vi "Host_GUI.vi"() -> ()   [LabVIEW 2017]
uses:
  <vilib>/Platform/TimedLoop/XDataNode/timing_clust.ctl
  <vilib>/Platform/TimedLoop/XDataNode/nitl_modes.ctl
  <vilib>/Platform/TimedLoop/XDataNode/wakeup.ctl
  <vilib>/Platform/TimedLoop/XDataNode/XDataNode.xnode
  <vilib>/FTP/NI_FTP.lvlib
  <vilib>/Platform/TimedLoop/XDataNode/XDNodeRunTimeDep.lvlib
panel:
  out "min index(es)":i32
  out "min value":dbl
  out "array":dbl[][](array[numeric])
  out "Enum":T1(ring)
  in  "Tab Control":T2(tab)
  in  "Initialization Parameters":T3={"W_b ini [rad/s]"=[0.0, 0.0, 0.0], "W ini [rad/s]"=[0.0, 0.0, 0.0], "altitude_ini(m)"=50.638, "lon_ini [º]"=-44.367775, "latd_ini [º]"=-2.3159948, "V_ini [m/s]"=[0.0, 0.0, 0.0], "Initial Euler Angles [deg]"=[0.0, 0.0, 0.0], "CFN-61G Enable"=FALSE, "Table enable"=FALSE, "DMARS Enable"=FALSE, "German TVA Enable"=FALSE, "Sim_Time [s]"=82.0, "Control Selection"=enum."Sim Control", "LOG Enable"=FALSE, "BR ACT enable"=FALSE} {"lon_ini [º]" format="%#_11g"; "latd_ini [º]" format="%#_10g"}
  in  "Simulation Parameters":T4={"Wind VelocityAzimuth [deg] "=0.0, "Wind Velocity Module [m/s]"=0.0, "Fe gain"=1.0, "Cnalpha gain"=1.0, "clp gain"=1.0, "cld gain"=1.0, "cmq gain"=1.0, "cnr gain"=1.0, "dl [º]"=0.0, "Nozzle misalignment yaw/pitch [º]"=[0.0, 0.0], "Nozzle eccentricity yaw/pitch [m]"=[], "Wind_Profile"=0} {"Wind_Profile" min=0 max=3 step=1; "Wind Velocity Module [m/s]" format="%#_13g"; "Wind VelocityAzimuth [deg]" format="%#_13g"}
  in  "Continuar":bool
  in  "stop":bool
  in  "Continuar":bool
  out "Table Monitor":T5(graph)
  out "OUTER":cluster{dbl, dbl, dbl} {"?" format="%1_6g"}
  out "INNER":cluster{dbl, dbl, dbl} {"?" format="%_6g"; "?" format="%#1_6g"}
  out "MIDDLE":cluster{dbl, dbl, dbl} {"?" format="%1_6g"}
  out "Euler Angles Simulation [deg]":T5(graph)
  in  "START_SIM":bool
  out "Sim_Stopped":bool
  in  "stop RT":bool
  out "Simulation time [s]":dbl
  out "Atitude":refnum<vi>(3d-picture)
  out "Altitude [m]":dbl
  out "Latitude/Longitude Sim [deg]":dbl[](array[numeric])
  out "Table ready":bool
  in  "Selector":enum16{"INNER", "MIDDLE", "OUTER"}(ring)=enum."OUTER"
  out "Euler Angles CFN [deg]":T5(graph)
  out "Euler Angles Diff (sim; INS)":cluster{dbl, dbl, dbl}
  out "Latitude/Longitude Ref [deg]":dbl[](array[numeric])
  out "Iteration Duration":i64
  out "Table Commands":T5(graph)
  in  "Selector 2":enum16{"INNER", "MIDDLE", "OUTER"}(ring)=enum."OUTER"
  out "Rates Sim [deg/s]":cluster{dbl, dbl, dbl}
  in  "Tab Control 2":T6(tab)
  out "Position":cluster{dbl[], dbl[]}[](graph)
  out "Velocity":cluster{dbl[], dbl[]}[](graph)
  out "Quaternions":cluster{dbl[], dbl[]}[](graph)
  out "Euler Angles":cluster{dbl[], dbl[]}[](graph)
  out "Body Rates":cluster{dbl[], dbl[]}[](graph)
  out "Body Accelerations":cluster{dbl[], dbl[]}[](graph)
  out "Malpha/ Mbeta":cluster{dbl[], dbl[]}[](graph)
  out "Angles of attack":cluster{dbl[], dbl[]}[](graph)
  out "ACT_b_angles":cluster{dbl[], dbl[]}[](graph)
  out "Oil Consumption":cluster{dbl[], dbl[]}(graph)
  out "Bending Moments":dbl[](graph)
  out "Guidance errors":cluster{dbl[], dbl[]}[](graph)
  out "Pos comparison":cluster{dbl[], dbl[]}[](graph)
  out "Euler Angles 2":cluster{dbl[], dbl[]}[](graph)
  out "file error":errorcluster
  # "POS"
  # "RATE"
  # "ACCEL"
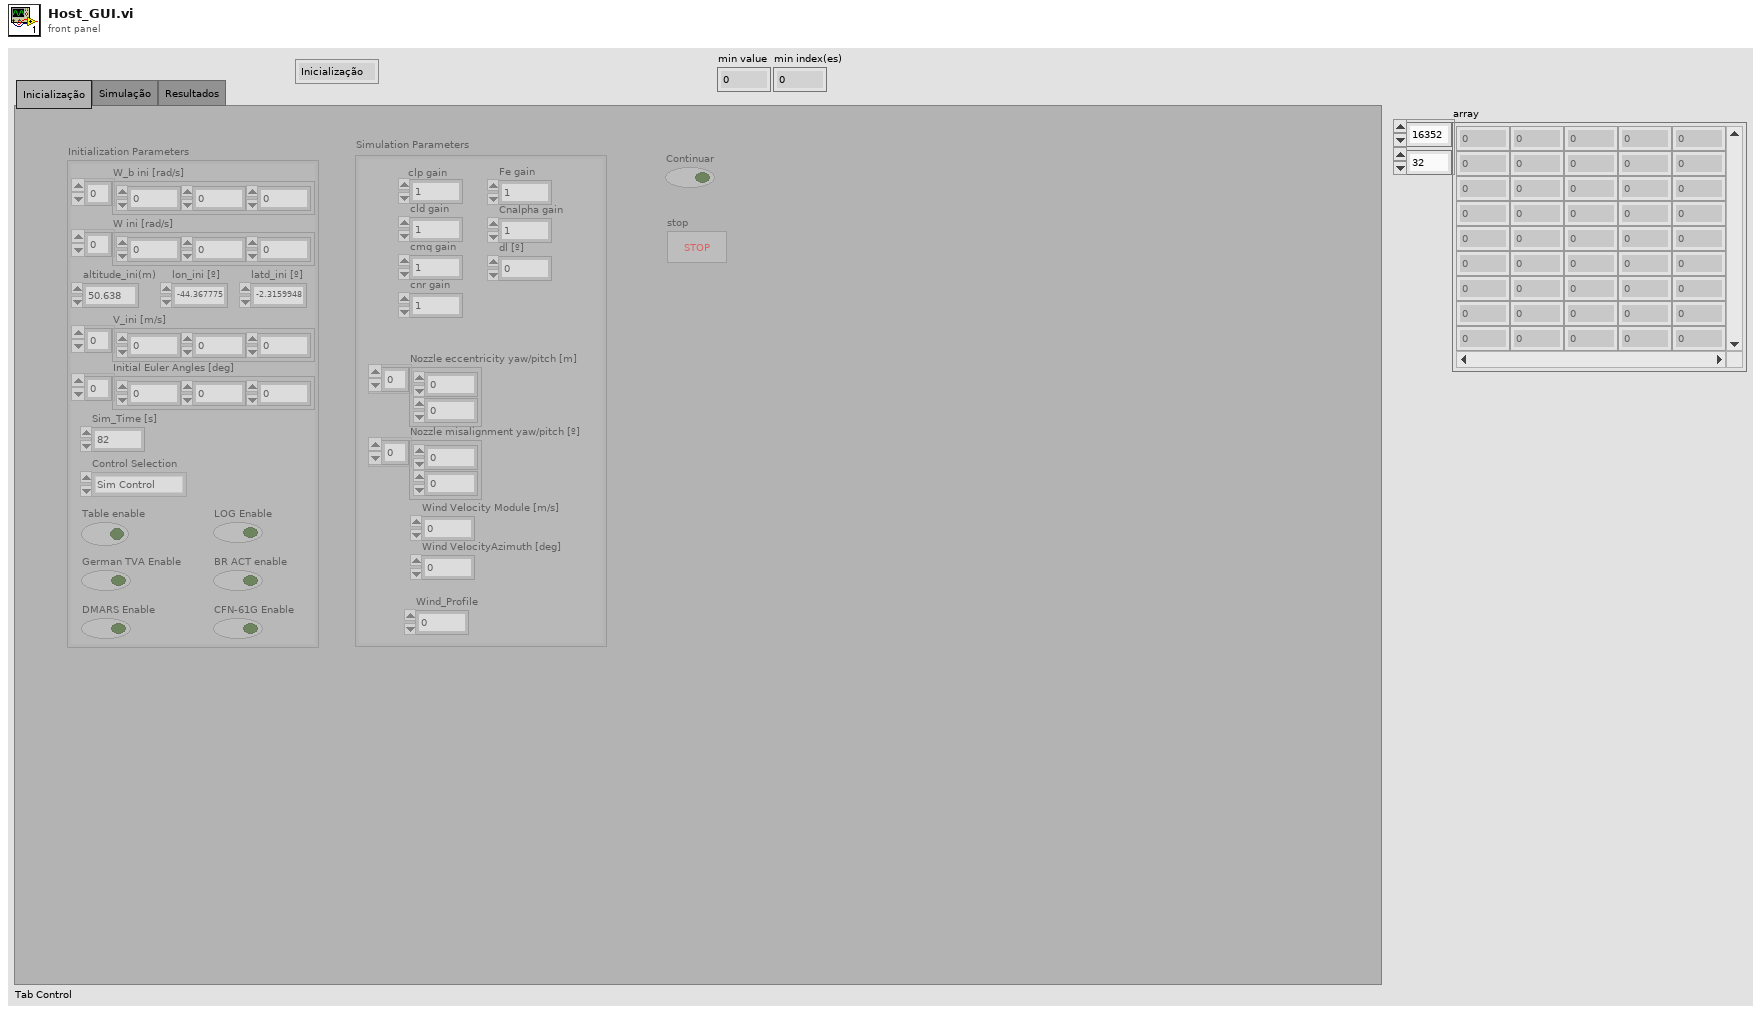
[diagram p1: front panel]
types:
  T1 = enum16{"Inicialização", "Simulação", "Resultados", "Finalizar RT"}
  T2 = enum32{"Inicialização", "Simulação", "Resultados"}
  T3 = cluster{"W_b ini [rad/s]":dbl[], "W ini [rad/s]":dbl[], "altitude_ini(m)":dbl, "lon_ini [º]":dbl, "latd_ini [º]":dbl, "V_ini [m/s]":dbl[], "Initial Euler Angles [deg]":dbl[], "CFN-61G Enable":bool, "Table enable":bool, "DMARS Enable":bool, "German TVA Enable":bool, "Sim_Time [s]":dbl, "Control Selection":enum16{"Constant", "TVA E-BOX", "Sim Control"}, "LOG Enable":bool, "BR ACT enable":bool}
  T4 = cluster{"Wind VelocityAzimuth [deg] ":dbl, "Wind Velocity Module [m/s]":dbl, "Fe gain":dbl, "Cnalpha gain":dbl, "clp gain":dbl, "cld gain":dbl, "cmq gain":dbl, "cnr gain":dbl, "dl [º]":dbl, "Nozzle misalignment yaw/pitch [º]":dbl[], "Nozzle eccentricity yaw/pitch [m]":dbl[], "Wind_Profile":i32}
  T5 = cluster{"Numeric":dbl, "Numeric":dbl, "Numeric":dbl}
  T6 = enum32{"Position", "Velocity", "Attitude Quaternions", "Attitude Euler Angles", "Body Rates", "Accel", "Malpha/ Mbeta", "AoA", "ACT_b angles", "Oil Consumption", "Bending Moments", "Guidance errors", "Position Comparison", "Attitude Comparison"}
  T7 = enum8{"Enabled", "Disabled", "Disabled and Grayed Out"}
  T8 = typedef "XDNodeRunTimeDep.lvlib/timing_clust.ctl" = cluster{"Expected End [f-1]":u64, "Actual End [f-1]":u64, "Finished Late? [f-1]":bool, "Expected End [i-1]":u64, "Actual End [i-1]":u64, "Finished Late? [i-1]":bool, "Expected Start [i]":u64, "Actual Start [i]":u64, "Expected Start [f]":u64, "Actual Start [f]":u64, "Source Name":string, "Structure Name":string, "Period":i64, "Deadline":i64, "Offset":i64, "Start":i64, "Priority":i32, "Timeout":i32, "Mode":T9, "Wakeup Reason":T10, "Error":errorcluster, "Source Type":string, "Secondary Source Type":string, "Global End Time":u64, "Global Start Time":u64, "Frame Duration":u64, "Iteration Duration":u64, "Assigned CPU":i32, "I/O Scan Engine Mode":u32}
  T9 = typedef "XDNodeRunTimeDep.lvlib/nitl_modes.ctl" = enum32{"No Change", "Process missed periods, maintain original phase", "Discard missed periods, maintain original phase", "Process missed periods, ignore original phase", "Discard missed periods, ignore original phase"}
  T10 = typedef "XDNodeRunTimeDep.lvlib/wakeup.ctl" = enum32{"Normal", "Aborted", "Asynchronous wakeup", "Timing source error", "Timed loop error", "Timeout"}
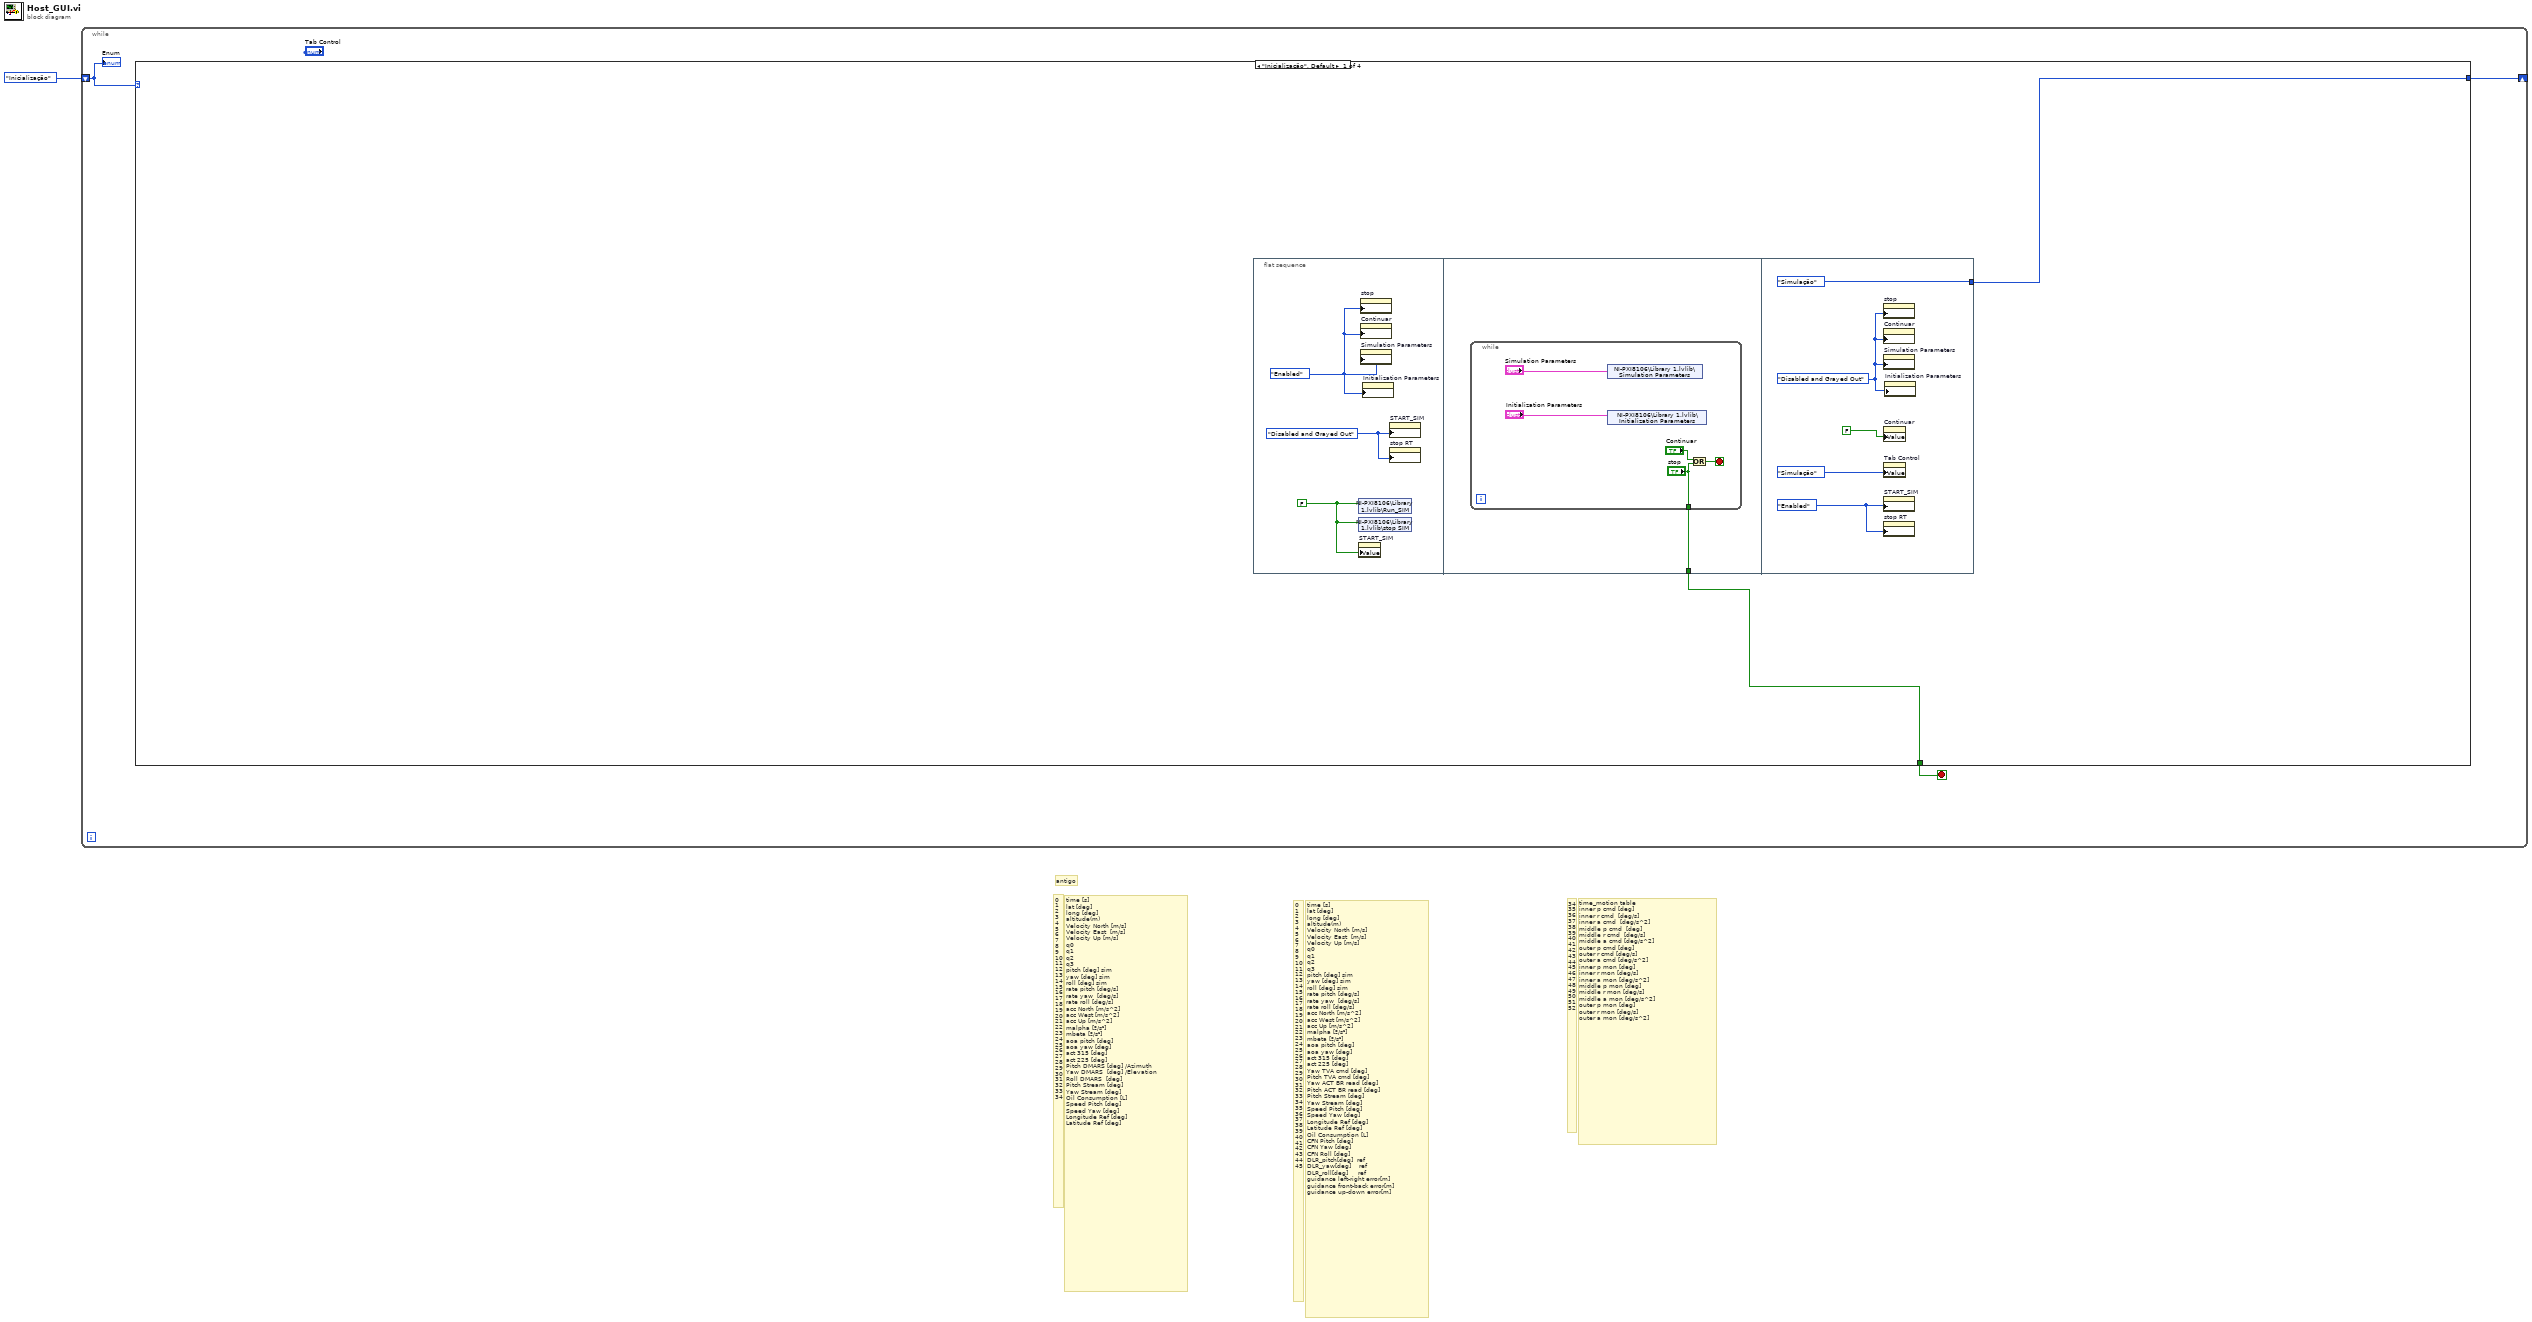
[diagram p0: block diagram]
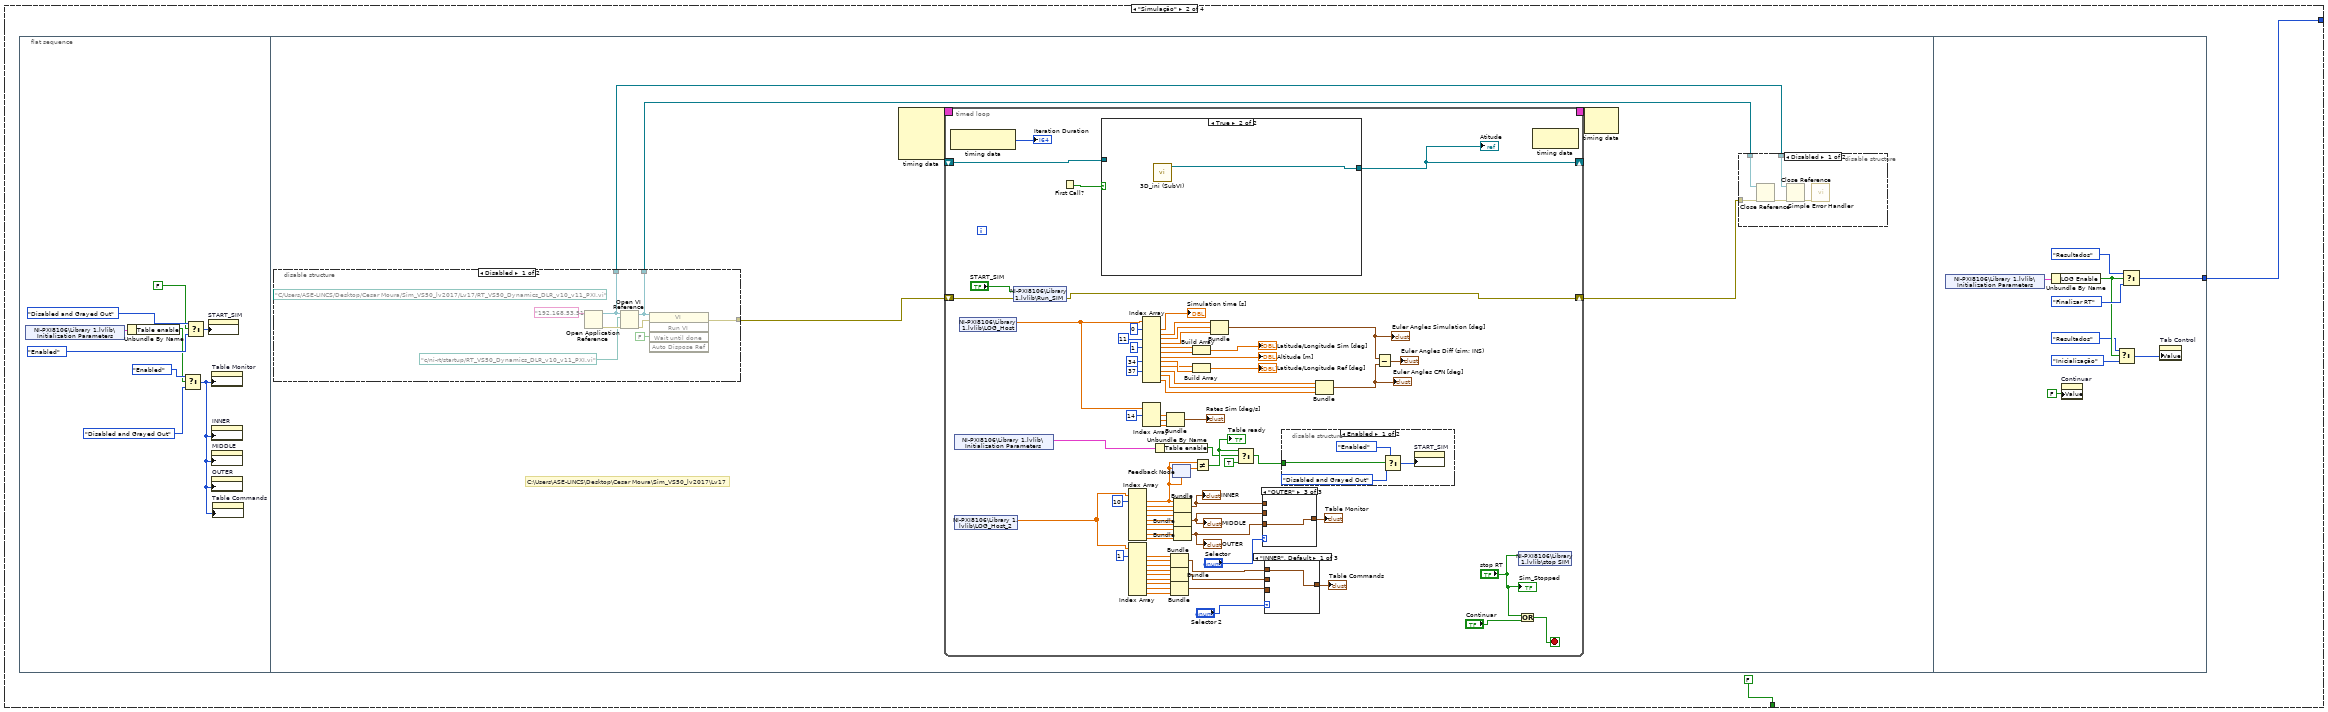
[diagram p2: hidden frame]
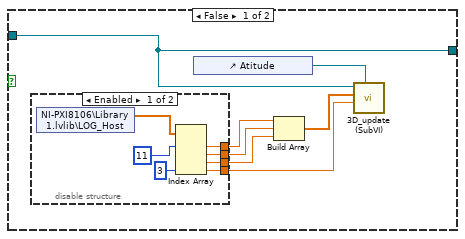
[diagram p8: hidden frame]
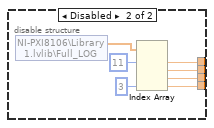
[diagram p9: hidden frame]
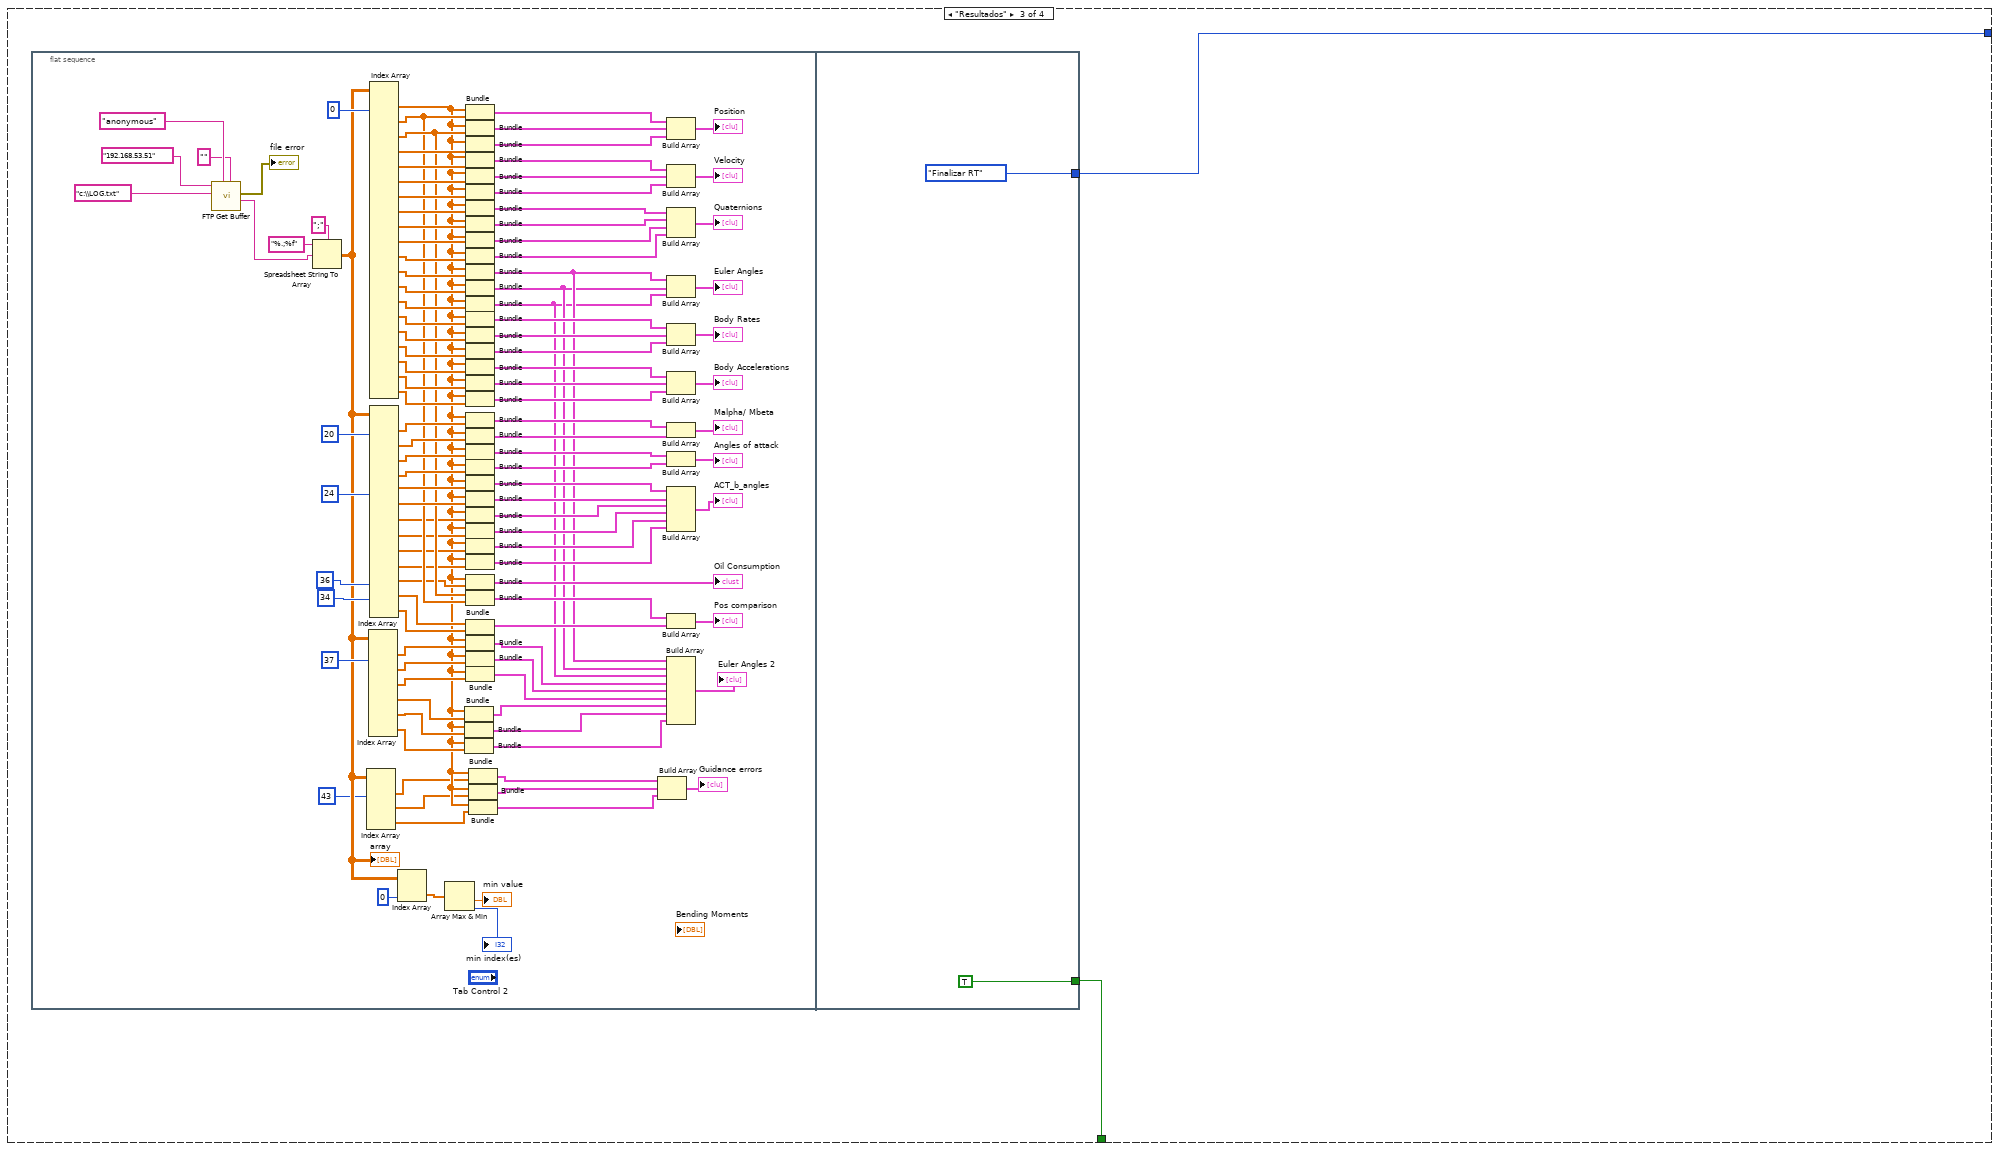
[diagram p12: hidden frame]
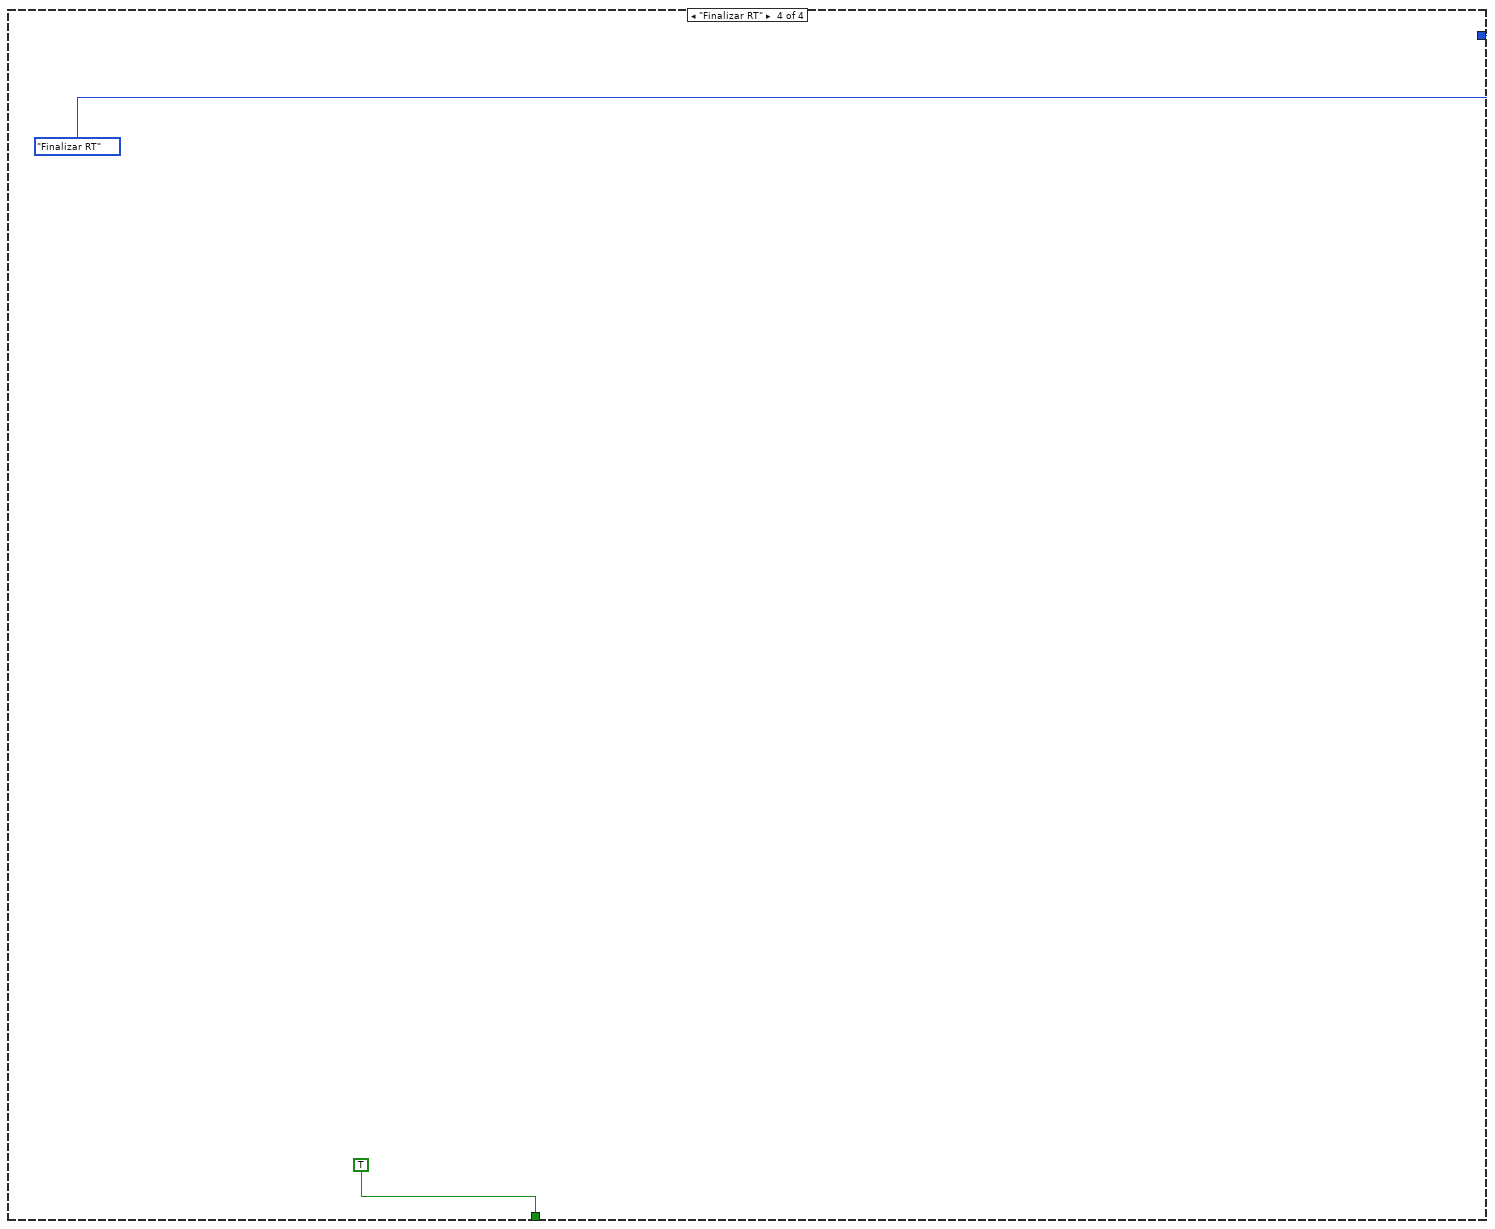
[diagram p13: hidden frame]
diagram:
  # "antigo"
  # "time [s]\nlat [deg]\nlong [deg]\naltitude(m)\nVelocity North [m/s]\nVelocity East  [m/s]\nVelocity Up [m/s]\nq0\nq1\nq2\nq3\npitch [deg] sim\nyaw [deg] sim\nroll [deg] sim\nrate pitch [deg/s] \nrate yaw  [deg/s]\nrate roll [deg/s]\nacc North [m/s^2] \nacc West [m/s^2]\nacc Up [m/s^2]\nmalpha [º/s²]\nmbeta [º/s²]\naoa pitch [deg] \naoa yaw [deg]\nact 315 [deg] \nact 225 [deg]\nYaw TVA cmd [deg]\nPitch TVA cmd [deg]\nYaw ACT BR read [deg]\nPitch ACT BR read [deg]\nPitch Stream [deg]\nYaw Stream [deg]\nSpeed Pitch [deg]\nSpeed Yaw [deg]\nLongitude Ref [deg]\nLatitude Ref [deg]\nOil Consumption [L]\nCFN Pitch [deg]\nCFN Yaw [deg]\nCFN Roll [deg]\nDLR_pitch[deg]  ref\nDLR_yaw[deg]    ref\nDLR_roll[deg]     ref\nguidance left-right error[m]\nguidance front-back error[m]\nguidance up-down error[m]"
  # "0\n1\n2\n3\n4\n5\n6\n7\n8\n9\n10\n11\n12\n13\n14\n15\n16\n17\n18\n19\n20\n21\n22\n23\n24\n25\n26\n27\n28\n29\n30\n31\n32\n33 34\n35\n36\n37\n38\n39\n40\n41\n42\n43\n44\n45"
  # "time_motion table\ninner p cmd [deg]\ninner r cmd  [deg/s]\ninner a cmd  [deg/s^2]\nmiddle p cmd  [deg]\nmiddle r cmd  [deg/s]\nmiddle a cmd [deg/s^2]\nouter p cmd [deg]\nouter r cmd [deg/s]\nouter a cmd [deg/s^2]\ninner p mon [deg]\ninner r mon [deg/s]\ninner a mon [deg/s^2]\nmiddle p mon [deg]\nmiddle r mon [deg/s]\nmiddle a mon [deg/s^2]\nouter p mon [deg]\nouter r mon [deg/s]\nouter a mon [deg/s^2]"
  # "34\n35\n36\n37\n38\n39\n40\n41\n42\n43\n44\n45\n46\n47\n48\n49\n50\n51\n52"
  # "0\n1\n2\n3\n4\n5\n6\n7\n8\n9\n10\n11\n12\n13\n14\n15\n16\n17\n18\n19\n20\n21\n22\n23\n24\n25\n26\n27\n28\n29\n30\n31\n32\n33 34"
  # "time [s]\nlat [deg]\nlong [deg]\naltitude(m)\nVelocity North [m/s]\nVelocity East  [m/s]\nVelocity Up [m/s]\nq0\nq1\nq2\nq3\npitch [deg] sim\nyaw [deg] sim\nroll [deg] sim\nrate pitch [deg/s] \nrate yaw  [deg/s]\nrate roll [deg/s]\nacc North [m/s^2] \nacc West [m/s^2]\nacc Up [m/s^2]\nmalpha [º/s²]\nmbeta [º/s²]\naoa pitch [deg] \naoa yaw [deg]\nact 315 [deg] \nact 225 [deg]\nPitch DMARS [deg] /Azimuth\nYaw DMARS  [deg] /Elevation\nRoll DMARS  [deg]\nPitch Stream [deg]\nYaw Stream [deg]\nOil Consumption [L]\nSpeed Pitch [deg]\nSpeed Yaw [deg]\nLongitude Ref [deg]\nLatitude Ref [deg]"
  n1 = while {
    shift-right: [w3] -> _
    shift-left: T1."Inicialização" -> [w4]
    stop <- w2 stop-if-true
    n2 = case shown="\"Inicialização\", Default" w4 {
      tunnel: [w6 w22 w173 T1."Finalizar RT"] -> w3
      tunnel: [w5 FALSE ("stop GUI") w172 TRUE ("stop GUI")] -> w2
      frame "Inicialização", Default {
        n3 = flat-sequence {
          tunnel: [w10] -> w5
          tunnel: [T1."Simulação"] -> w6
          frame #0 {
            w8 = T7."Disabled and Grayed Out" ("Disabled")
            w9 = FALSE ("Run_SIM")
            w7 = T7."Enabled" ("Disabled")
            n4 = shared-variable "NI-PXI8106\\Library 1.lvlib\\Run_SIM"(w9) -> ()  [unwired: 1 in, 1 out]
            n5 = shared-variable "NI-PXI8106\\Library 1.lvlib\\stop SIM"(w9) -> ()  [unwired: 1 in, 1 out]
            n6 = property on="START_SIM" class="Bool (strict)"("Value"=w9) -> ()  [unwired: 2 in, 2 out]
            n7 = property on="stop" class="Bool"("DisabledEnum"=w7) -> ()  [unwired: 2 in, 2 out]
            n8 = property on="Continuar" class="Bool (strict)"("DisabledEnum"=w7) -> ()  [unwired: 2 in, 2 out]
            n9 = property on="Simulation Parameters" class="Clust (strict)"("DisabledEnum"=w7) -> ()  [unwired: 2 in, 2 out]
            n10 = property on="Initialization Parameters" class="Clust (strict)"("DisabledEnum"=w7) -> ()  [unwired: 2 in, 2 out]
            n11 = property on="START_SIM" class="Bool (strict)"("DisabledEnum"=w8) -> ()  [unwired: 2 in, 2 out]
            n12 = property on="stop RT" class="Bool"("DisabledEnum"=w8) -> ()  [unwired: 2 in, 2 out]
          }
          frame #1 {
            n13 = while {
              tunnel: ["stop"] -> w10
              stop <- w12 stop-if-true
              n14 = shared-variable "NI-PXI8106\\Library 1.lvlib\\Simulation Parameters"("Simulation Parameters") -> ()  [unwired: 1 in, 1 out]
              n15 = shared-variable "NI-PXI8106\\Library 1.lvlib\\Initialization Parameters"("Initialization Parameters") -> ()  [unwired: 1 in, 1 out]
              n16 = Or(x="Continuar", y="stop") -> (x .or. y?=w12:bool)
            }
          }
          frame #2 {
            w17 = T7."Enabled" ("Disabled")
            w16 = T7."Disabled and Grayed Out" ("Disabled")
            n17 = property on="stop" class="Bool"("DisabledEnum"=w16) -> ()  [unwired: 2 in, 2 out]
            n18 = property on="Continuar" class="Bool (strict)"("DisabledEnum"=w16) -> ()  [unwired: 2 in, 2 out]
            n19 = property on="Simulation Parameters" class="Clust (strict)"("DisabledEnum"=w16) -> ()  [unwired: 2 in, 2 out]
            n20 = property on="Continuar" class="Bool (strict)"("Value"=FALSE ("Continuar")) -> ()  [unwired: 2 in, 2 out]
            n21 = property on="Tab Control" class="TabCtl (strict)"("Value"=enum32{"Inicialização", "Simulação"}."Simulação" ("Tab Control")) -> ()  [unwired: 2 in, 2 out]
            n22 = property on="START_SIM" class="Bool (strict)"("DisabledEnum"=w17) -> ()  [unwired: 2 in, 2 out]
            n23 = property on="stop RT" class="Bool"("DisabledEnum"=w17) -> ()  [unwired: 2 in, 2 out]
            n24 = property on="Initialization Parameters" class="Clust (strict)"("DisabledEnum"=w16) -> ()  [unwired: 2 in, 2 out]
          }
        }
      }
      frame "Simulação" {
        n25 = flat-sequence {
          tunnel: [w170] -> w22
          frame #0 {
            n26 = shared-variable "NI-PXI8106\\Library 1.lvlib\\Initialization Parameters"() -> (w31:T3)  [unwired: 1 in, 1 out]
            n27 = Unbundle By Name(w31) -> ("Table enable"=w25:bool)
            n28 = Select(t=T7."Enabled" ("Disabled"), s=w25, f=T7."Disabled and Grayed Out" ("Disabled")) -> (s? t:f=w23:T7)
            n29 = Select(t=T7."Disabled and Grayed Out" ("Disabled"), s=FALSE, f=T7."Enabled" ("Disabled")) -> (s? t:f=w28:T7)
            n30 = property on="START_SIM" class="Bool (strict)"("DisabledEnum"=w28) -> ()  [unwired: 2 in, 2 out]
            n31 = property on="Table Monitor" class="WFChart (strict)"("DisabledEnum"=w23) -> ()  [unwired: 2 in, 2 out]
            n32 = property on="INNER" class="Clust (strict)"("DisabledEnum"=w23) -> ()  [unwired: 2 in, 2 out]
            n33 = property on="MIDDLE" class="Clust (strict)"("DisabledEnum"=w23) -> ()  [unwired: 2 in, 2 out]
            n34 = property on="OUTER" class="Clust (strict)"("DisabledEnum"=w23) -> ()  [unwired: 2 in, 2 out]
            n35 = property on="Table Commands" class="WFChart (strict)"("DisabledEnum"=w23) -> ()  [unwired: 2 in, 2 out]
          }
          frame #1 {
            # "C:\\Users\\ASE-LINCS\\Desktop\\Cesar Moura\\Sim_VS50_lv2017\\Lv17"
            n36 = disable-structure shown="Disabled" {
              disable-tunnel: [w157 _] -> w35
              disable-tunnel: [w156 _] -> w37
              disable-tunnel: [w155 _] -> w36
              frame Disabled {
                (unwired) path "C:/Users/ASE-LINCS/Desktop/Cesar Moura/Sim_VS50_lv2017/Lv17/RT_VS50_Dynamics_DLR_v10_v11_PXI.vi" ("vi path")
                n37 = Open Application Reference(11:"192.168.53.51" ("machine name (\"\":  open local reference)")) -> (0:w153:errorcluster, 3:w155:refnum<vi>)  [unwired: 3 in]
                n38 = Open VI Reference(application reference (local)=w155, vi path=path "c:/ni-rt/startup/RT_VS50_Dynamics_DLR_v10_v11_PXI.vi", error in (no error)=w153) -> (vi reference=w156:refnum<vi>, error out=w152:errorcluster)  [unwired: 3 in]
                n39 = invoke class="VI" method="Run VI"(reference=w156, error in=w152, "Wait until done"=FALSE ("Wait Until Done")) -> (error out=w157:errorcluster)  [unwired: 2 in, 4 out]
              }
              frame Enabled {
              }
            }
            n40 = node-c288() -> (w33:T8)  [unwired: 4 in]
            n41 = timed-loop {
              shift-right: [w111] -> _
              shift-left: _ -> [w112]
              shift-right: [w72] -> w34
              shift-left: w35 -> [w73]
              timing: w33 -> [_]
              timing-out: [_] -> w32
              stop <- w45 stop-if-true
              n42 = node-c288() -> (→"Iteration Duration":i64)  [unwired: 1 in]
              n43 = shared-variable "NI-PXI8106\\Library 1.lvlib\\Initialization Parameters"() -> (w103:T3)  [unwired: 1 in, 1 out]
              n44 = shared-variable "NI-PXI8106\\Library 1.lvlib\\LOG_Host_2"() -> (w54:dbl[])  [unwired: 1 in, 1 out]
              n45 = shared-variable "NI-PXI8106\\Library 1.lvlib\\LOG_Host"() -> (w43:dbl[])  [unwired: 1 in, 1 out]
              n46 = shared-variable "NI-PXI8106\\Library 1.lvlib\\Run_SIM"("START_SIM", error in=w73) -> (error out=w72:errorcluster)
              n47 = First Call?() -> (First Call?: T/F=w110:bool)
              n48 = case shown="True" w110 {
                tunnel: [w132 w147] -> w111
                tunnel: w112 -> [w132 _]
                frame False {
                  n49 = disable-structure shown="Enabled" {
                    disable-tunnel: [w136 w143] -> w130
                    disable-tunnel: [w135 w142] -> w129
                    disable-tunnel: [w134 w141] -> w128
                    disable-tunnel: [w133 w140] -> w126
                    frame Enabled {
                      n50 = shared-variable "NI-PXI8106\\Library 1.lvlib\\LOG_Host"() -> (w139:dbl[])  [unwired: 1 in, 1 out]
                      n51 = Index Array(array=w139, index #1=11 ("index"), index #4=3 ("index")) -> (element #1=w136:dbl, element #2=w135:dbl, element #3=w134:dbl, element #4=w133:dbl)  [unwired: 2 in]
                    }
                    frame Disabled {
                      n52 = shared-variable "NI-PXI8106\\Library 1.lvlib\\Full_LOG"() -> (w146:dbl[])  [unwired: 1 in, 1 out]
                      n53 = Index Array(array=w146, index #1=11 ("index"), index #4=3 ("index")) -> (element #1=w143:dbl, element #2=w142:dbl, element #3=w141:dbl, element #4=w140:dbl)  [unwired: 2 in]
                    }
                  }
                  n54 = control-ref of="Atitude"() -> (w127:refnum<vi>)
                  n55 = Build Array(w130, w129, w128) -> (w131:dbl[])
                  n56 = call "3D_update (SubVI).vi"("SceneGraphDisp Refnum"=w127, "Altitude [m]"=w126, "Euler Angles [deg]"=w131, "SceneObject in"=w132) -> ()  [unwired: 8 in]
                }
                frame True {
                  n57 = call "3D_ini (SubVI).vi"() -> ("SceneObject out"=w147:refnum<vi>)  [unwired: 11 in]
                }
              }
              "Atitude" <- w111
              n58 = Index Array(array=w54, index #1=10 ("index")) -> (element #1=w89:dbl, element #2=w90:dbl, element #3=w91:dbl, element #4=w92:dbl, element #5=w93:dbl, element #6=w94:dbl, element #7=w95:dbl, element #8=w96:dbl, element #9=w97:dbl)  [unwired: 8 in]
              n59 = Index Array(array=w54, index #1=1 ("index")) -> (element #1=w70:dbl, element #2=w69:dbl, element #3=w68:dbl, element #4=w67:dbl, element #5=w66:dbl, element #6=w65:dbl, element #7=w64:dbl, element #8=w63:dbl, element #9=w62:dbl)  [unwired: 8 in]
              n60 = Index Array(array=w43, index #1=14 ("index")) -> (element #1=w42:dbl, element #2=w41:dbl, element #3=w40:dbl)  [unwired: 2 in]
              n61 = Index Array(array=w43, index #1=0 ("index"), index #2=11 ("index"), index #5=1 ("index"), index #8=34 ("index"), index #10=37 ("index")) -> (element #1=→"Simulation time [s]":dbl, element #2=w82:dbl, element #3=w83:dbl, element #4=w84:dbl, element #5=w85:dbl, element #6=w86:dbl, element #7=→"Altitude [m]":dbl, element #8=w48:dbl, element #9=w47:dbl, element #10=w51:dbl, element #11=w50:dbl, element #12=w49:dbl)  [unwired: 7 in]
              n62 = Unbundle By Name(w103) -> ("Table enable"=w104:bool)
              n63 = Bundle("Numeric"=w42, "Numeric"=w41, "Numeric"=w40) -> (→"Rates Sim [deg/s]":T5)  [unwired: 1 in]
              n64 = Bundle("Numeric"=w70, "Numeric"=w69, "Numeric"=w68) -> (w61:T5)  [unwired: 1 in]
              n65 = Bundle("Numeric"=w67, "Numeric"=w66, "Numeric"=w65) -> (w60:T5)  [unwired: 1 in]
              n66 = Bundle("Numeric"=w64, "Numeric"=w63, "Numeric"=w62) -> (w57:T5)  [unwired: 1 in]
              n67 = feedback #1(w89) -> (w88:dbl)
              n68 = feedback-in #1(w89) -> ()
              n69 = Bundle("Numeric"=w89, "Numeric"=w90, "Numeric"=w91) -> (w100:T5)  [unwired: 1 in]
              "INNER" <- w100
              n70 = Bundle("Numeric"=w92, "Numeric"=w93, "Numeric"=w94) -> (w101:T5)  [unwired: 1 in]
              "MIDDLE" <- w101
              n71 = Bundle("Numeric"=w95, "Numeric"=w96, "Numeric"=w97) -> (w102:T5)  [unwired: 1 in]
              "OUTER" <- w102
              n72 = Build Array(w85, w86) -> (→"Latitude/Longitude Sim [deg]":dbl[])
              n73 = Build Array(w47, w48) -> (→"Latitude/Longitude Ref [deg]":dbl[])
              n74 = Not Equal?(x=w89, y=w88) -> (x != y?=w108:bool)
              "Table ready" <- w108
              n75 = Bundle("Numeric"=w82, "Numeric"=w83, "Numeric"=w84) -> (w87:T5)  [unwired: 1 in]
              "Euler Angles Simulation [deg]" <- w87
              n76 = Select(t=w108, s=w104, f=TRUE) -> (s? t:f=w105:bool)
              n77 = case shown="\"OUTER\"" "Selector" {
                tunnel: [w123 w124 w125] -> w99
                tunnel: w100 -> [w123 _ _]
                tunnel: w101 -> [_ w124 _]
                tunnel: w102 -> [_ _ w125]
                frame "INNER", Default {
                }
                frame "MIDDLE" {
                }
                frame "OUTER" {
                }
              }
              "Table Monitor" <- w99
              n78 = case shown="\"INNER\", Default" "Selector 2" {
                tunnel: [w113 w114 w115] -> w58
                tunnel: w61 -> [w113 _ _]
                tunnel: w60 -> [_ w114 _]
                tunnel: w57 -> [_ _ w115]
                frame "INNER", Default {
                }
                frame "MIDDLE" {
                }
                frame "OUTER" {
                }
              }
              "Table Commands" <- w58
              n79 = disable-structure shown="Enabled" {
                disable-tunnel: w105 -> [w118 _]
                frame Enabled {
                  n80 = Select(t=T7."Enabled" ("Disabled"), s=w118, f=T7."Disabled and Grayed Out" ("Disabled")) -> (s? t:f=w119:T7)
                  n81 = property on="START_SIM" class="Bool (strict)"("DisabledEnum"=w119) -> ()  [unwired: 2 in, 2 out]
                }
                frame Disabled {
                }
              }
              n82 = Bundle("Numeric"=w51, "Numeric"=w50, "Numeric"=w49) -> (w78:T5)  [unwired: 1 in]
              "Euler Angles CFN [deg]" <- w78
              n83 = Subtract(x=w87, y=w78) -> (x-y=→"Euler Angles Diff (sim; INS)":T5)
              n84 = shared-variable "NI-PXI8106\\Library 1.lvlib\\stop SIM"("stop RT") -> ()  [unwired: 1 in, 1 out]
              n85 = Or(x="stop RT", y="Continuar") -> (x .or. y?=w45:bool)
              n86 = node-c288() -> ()  [unwired: 1 in, 1 out]
              "Sim_Stopped" <- "stop RT"
            }
            n87 = node-c288(w32) -> ()  [unwired: 1 out]
            n88 = disable-structure shown="Disabled" {
              disable-tunnel: w37 -> [w162 _]
              disable-tunnel: w36 -> [w161 _]
              disable-tunnel: w34 -> [w158 _]
              frame Disabled {
                n89 = Close Reference(reference=w162, error in (no error)=w158) -> (error out=w160:errorcluster)
                n90 = Close Reference(reference=w161, error in (no error)=w160) -> (error out=w159:errorcluster)
                n91 = call <vilib>:"Simple Error Handler.vi"("error in (no error)"=w159) -> ()  [unwired: 4 in, 5 out]
              }
              frame Enabled {
              }
            }
          }
          frame #2 {
            n92 = shared-variable "NI-PXI8106\\Library 1.lvlib\\Initialization Parameters"() -> (w171:T3)  [unwired: 1 in, 1 out]
            n93 = Unbundle By Name(w171) -> ("LOG Enable"=w166:bool)
            n94 = property on="Continuar" class="Bool (strict)"("Value"=FALSE ("Continuar 2")) -> ()  [unwired: 2 in, 2 out]
            n95 = Select(t=T2."Resultados" ("Tab Control"), s=w166, f=T2."Inicialização") -> (s? t:f=w164:T2)
            n96 = Select(t=T1."Resultados", s=w166, f=T1."Finalizar RT") -> (s? t:f=w170:T1)
            n97 = property on="Tab Control" class="TabCtl (strict)"("Value"=w164) -> ()  [unwired: 2 in, 2 out]
          }
        }
      }
      frame "Resultados" {
        n98 = flat-sequence {
          tunnel: [T1."Finalizar RT"] -> w173
          tunnel: [TRUE ("stop GUI 2")] -> w172
          frame #0 {
            n99 = call <vilib>:"FTP Get Buffer.vi"("password"="", "user"="anonymous", "remote path"="c:\\LOG.txt", "host"="192.168.53.51") -> ("data"=w282:string, "file error"=→"file error":errorcluster)  [unwired: 5 in, 1 out]
            n100 = Spreadsheet String To Array(delimiter (Tab)=";", format string="%.;%f", spreadsheet string=w282) -> (array=w182:dbl[][])  [unwired: 1 in]
            "array" <- w182
            n101 = Index Array(array=w182, index (col) #1=43 ("disabled index (col)")) -> (element #1=w179:dbl[], element #2=w178:dbl[], element #3=w177:dbl[])  [unwired: 5 in]
            n102 = Index Array(array=w182, index (col) #1=37 ("index (col)")) -> (element #1=w196:dbl[], element #2=w195:dbl[], element #3=w194:dbl[], element #4=w189:dbl[], element #5=w188:dbl[], element #6=w187:dbl[])  [unwired: 11 in]
            n103 = Index Array(array=w182, index (col) #1=0 ("index (row)")) -> (element #1=w180:dbl[], element #2=w222:dbl[], element #3=w223:dbl[], element #4=w227:dbl[], element #5=w274:dbl[], element #6=w273:dbl[], element #7=w272:dbl[], element #8=w266:dbl[], element #9=w265:dbl[], element #10=w264:dbl[], element #11=w263:dbl[], element #12=w261:dbl[], element #13=w260:dbl[], element #14=w259:dbl[], element #15=w252:dbl[], element #16=w253:dbl[], element #17=w254:dbl[], element #18=w247:dbl[], element #19=w246:dbl[], element #20=w245:dbl[])  [unwired: 39 in]
            n104 = Index Array(array=w182, index (col) #1=20 ("disabled index (col)"), index (col) #5=24 ("index (col)"), index (col) #11=36 ("index (col)"), index (col) #12=34 ("index (col)")) -> (element #1=w240:dbl[], element #2=w239:dbl[], element #3=w235:dbl[], element #4=w234:dbl[], element #5=w230:dbl[], element #6=w229:dbl[], element #7=w213:dbl[], element #8=w212:dbl[], element #9=w204:dbl[], element #10=w203:dbl[], element #11=w205:dbl[], element #12=w206:dbl[], element #13=w207:dbl[])  [unwired: 22 in]
            n105 = Index Array(array=w182, index (col)=0 ("disabled index (col)")) -> (element=w220:dbl[])  [unwired: 1 in]
            n106 = Array Max & Min(array=w220) -> (min value=→"min value":dbl, min index (indices)=→"min index(es)":i32)  [unwired: 2 out]
            n107 = Bundle(w180, w189) -> (w184:cluster{dbl[], dbl[]})  [unwired: 1 in]
            n108 = Bundle(w180, w188) -> (w185:cluster{dbl[], dbl[]})  [unwired: 1 in]
            n109 = Bundle(w180, w187) -> (w186:cluster{dbl[], dbl[]})  [unwired: 1 in]
            n110 = Bundle(w180, w222) -> (w224:cluster{dbl[], dbl[]})  [unwired: 1 in]
            n111 = Bundle(w180, w223) -> (w226:cluster{dbl[], dbl[]})  [unwired: 1 in]
            n112 = Bundle(w180, w227) -> (w225:cluster{dbl[], dbl[]})  [unwired: 1 in]
            n113 = Bundle(w180, w274) -> (w276:cluster{dbl[], dbl[]})  [unwired: 1 in]
            n114 = Bundle(w180, w273) -> (w277:cluster{dbl[], dbl[]})  [unwired: 1 in]
            n115 = Bundle(w180, w272) -> (w278:cluster{dbl[], dbl[]})  [unwired: 1 in]
            n116 = Bundle(w180, w266) -> (w269:cluster{dbl[], dbl[]})  [unwired: 1 in]
            n117 = Bundle(w180, w265) -> (w271:cluster{dbl[], dbl[]})  [unwired: 1 in]
            n118 = Bundle(w180, w264) -> (w270:cluster{dbl[], dbl[]})  [unwired: 1 in]
            n119 = Bundle(w180, w263) -> (w268:cluster{dbl[], dbl[]})  [unwired: 1 in]
            n120 = Bundle(w180, w261) -> (w199:cluster{dbl[], dbl[]})  [unwired: 1 in]
            n121 = Bundle(w180, w260) -> (w198:cluster{dbl[], dbl[]})  [unwired: 1 in]
            n122 = Bundle(w180, w259) -> (w197:cluster{dbl[], dbl[]})  [unwired: 1 in]
            n123 = Bundle(w180, w252) -> (w258:cluster{dbl[], dbl[]})  [unwired: 1 in]
            n124 = Bundle(w180, w253) -> (w257:cluster{dbl[], dbl[]})  [unwired: 1 in]
            n125 = Bundle(w180, w254) -> (w256:cluster{dbl[], dbl[]})  [unwired: 1 in]
            n126 = Bundle(w180, w247) -> (w250:cluster{dbl[], dbl[]})  [unwired: 1 in]
            n127 = Bundle(w180, w246) -> (w249:cluster{dbl[], dbl[]})  [unwired: 1 in]
            n128 = Bundle(w180, w245) -> (w248:cluster{dbl[], dbl[]})  [unwired: 1 in]
            n129 = Bundle(w180, w240) -> (w244:cluster{dbl[], dbl[]})  [unwired: 1 in]
            n130 = Bundle(w180, w239) -> (w243:cluster{dbl[], dbl[]})  [unwired: 1 in]
            n131 = Bundle(w180, w235) -> (w236:cluster{dbl[], dbl[]})  [unwired: 1 in]
            n132 = Bundle(w180, w234) -> (w238:cluster{dbl[], dbl[]})  [unwired: 1 in]
            n133 = Bundle(w180, w230) -> (w232:cluster{dbl[], dbl[]})  [unwired: 1 in]
            n134 = Bundle(w180, w229) -> (w233:cluster{dbl[], dbl[]})  [unwired: 1 in]
            n135 = Bundle(w180, w213) -> (w210:cluster{dbl[], dbl[]})  [unwired: 1 in]
            n136 = Bundle(w180, w212) -> (w211:cluster{dbl[], dbl[]})  [unwired: 1 in]
            n137 = Bundle(w180, w204) -> (w201:cluster{dbl[], dbl[]})  [unwired: 1 in]
            n138 = Bundle(w180, w203) -> (w202:cluster{dbl[], dbl[]})  [unwired: 1 in]
            n139 = Bundle(w180, w205) -> (→"Oil Consumption":cluster{dbl[], dbl[]})  [unwired: 1 in]
            n140 = Bundle(w223, w222) -> (w217:cluster{dbl[], dbl[]})  [unwired: 1 in]
            n141 = Bundle(w206, w207) -> (w216:cluster{dbl[], dbl[]})  [unwired: 1 in]
            n142 = Bundle(w180, w196) -> (w192:cluster{dbl[], dbl[]})  [unwired: 1 in]
            n143 = Bundle(w180, w195) -> (w191:cluster{dbl[], dbl[]})  [unwired: 1 in]
            n144 = Bundle(w180, w194) -> (w193:cluster{dbl[], dbl[]})  [unwired: 1 in]
            n145 = Bundle(w180, w179) -> (w176:cluster{dbl[], dbl[]})  [unwired: 1 in]
            n146 = Bundle(w180, w178) -> (w175:cluster{dbl[], dbl[]})  [unwired: 1 in]
            n147 = Bundle(w180, w177) -> (w174:cluster{dbl[], dbl[]})  [unwired: 1 in]
            n148 = Build Array(w176, w175, w174) -> (→"Guidance errors":cluster{dbl[], dbl[]}[])
            n149 = Build Array(w224, w226, w225) -> (→"Position":cluster{dbl[], dbl[]}[])
            n150 = Build Array(w276, w277, w278) -> (→"Velocity":cluster{dbl[], dbl[]}[])
            n151 = Build Array(w269, w271, w270, w268) -> (→"Quaternions":cluster{dbl[], dbl[]}[])
            n152 = Build Array(w199, w198, w197) -> (→"Euler Angles":cluster{dbl[], dbl[]}[])
            n153 = Build Array(w258, w257, w256) -> (→"Body Rates":cluster{dbl[], dbl[]}[])
            n154 = Build Array(w250, w249, w248) -> (→"Body Accelerations":cluster{dbl[], dbl[]}[])
            n155 = Build Array(w244, w243) -> (→"Malpha/ Mbeta":cluster{dbl[], dbl[]}[])
            n156 = Build Array(w236, w238) -> (→"Angles of attack":cluster{dbl[], dbl[]}[])
            n157 = Build Array(w232, w233, w210, w211, w201, w202) -> (→"ACT_b_angles":cluster{dbl[], dbl[]}[])
            n158 = Build Array(w217, w216) -> (→"Pos comparison":cluster{dbl[], dbl[]}[])
            n159 = Build Array(w199, w198, w197, w192, w191, w193, w184, w185, w186) -> (→"Euler Angles 2":cluster{dbl[], dbl[]}[])
          }
          frame #1 {
          }
        }
      }
      frame "Finalizar RT" {
      }
    }
    "Enum" <- w4
  }
